vi "Send Event.vi"(10 "Data":variant, 11 "LINX Shortcut":T1) -> ()   [LabVIEW 2019, in "LINX.lvlib" / "LINX.lvclass"]
uses:
  LINX.lvclass
  LINX Shortcut.ctl
  Packed Libraries/Messaging.lvlibp/Message Cluster.ctl
  Packed Libraries/Messaging.lvlibp
  LINX Channel Type.ctl
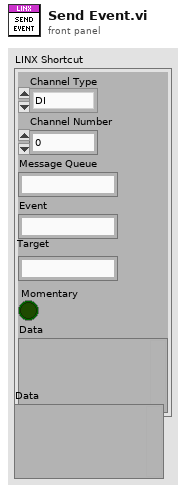
[diagram p1: front panel]
types:
  T1 = typedef "LINX.lvlib/LINX.lvclass/LINX Shortcut.ctl" = cluster{"Channel Type":T2, "Channel Number":u8, "Message Queue":string, "Event":string, "Target":string, "Momentary":bool, "Data":variant}
  T2 = typedef "LINX.lvlib/LINX.lvclass/LINX Channel Type.ctl" = enum16{"DI", "AI"}
  T3 = typedef "Messaging.lvlibp/Message Cluster.ctl" = cluster{"Event":string, "Source":string, "Target":string, "Data":variant}
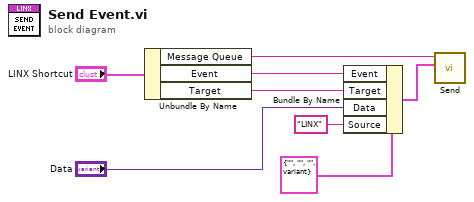
[diagram p0: block diagram]
diagram:
  n1 = Unbundle By Name("LINX Shortcut") -> ("Message Queue"=w8:string, "Event"=w5:string, "Target"=w4:string)
  n2 = Bundle By Name(cluster=T3 {"Event"="", "Source"="", "Target"="", "Data"=variant} ("Message"), "Event"=w5, "Target"=w4, "Data"="Data", "Source"="LINX") -> (w6:T3)
  n3 = call "Send.vi"("Message"=w6, "Queue Name"=w8) -> ()  [unwired: 9 in, 1 out]
